vi "DAQmx.Prime AO.vi"(8 "error in (no error)":errorcluster, 11 "DAQmx in":refnum<class "DAQmx.lvclass">) -> (0 "error out":errorcluster, 3 "DAQmx out":refnum<class "DAQmx.lvclass">)   [LabVIEW 2019, in "DAQmx.lvclass"]
uses:
  DAQmx.lvclass
  DAQmx.lvclass/DAQmx.ctl
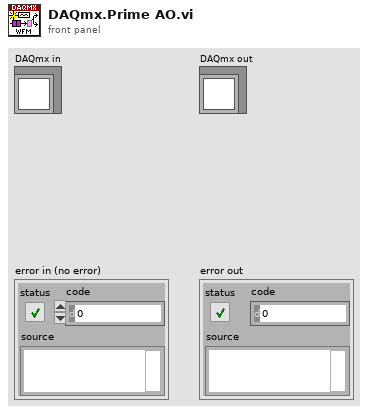
[diagram p1: front panel]
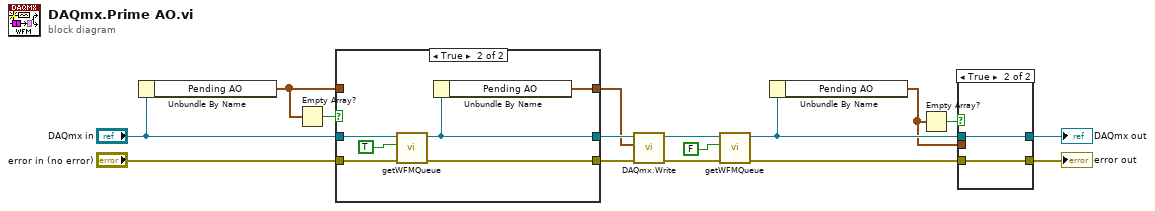
[diagram p0: block diagram]
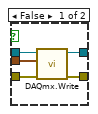
[diagram p2: hidden frame]
diagram:
  n1 = Unbundle By Name("DAQmx in") -> ("Pending AO"=w12:waveform(dbl)[])
  n2 = Empty Array?(array=w12) -> (empty?=w13:bool)
  n3 = case shown="True" w13 {
    tunnel: [w18 w21] -> w6
    tunnel: "DAQmx in" -> [w18 w25]
    tunnel: "error in (no error)" -> [w19 w24]
    tunnel: [w17 w20] -> w3
    tunnel: [w19 w22] -> w7
    tunnel: w12 -> [w17 _]
    frame False {
    }
    frame True {
      n4 = call "getWFMQueue.vi"("error in (no error)"=w24, "wait for min buffer?"=TRUE, "DAQmx in"=w25) -> ("error out"=w22:errorcluster, "DAQmx out"=w21:refnum<class "DAQmx.lvclass">)  [unwired: 6 in, 1 out]
      n5 = Unbundle By Name(w21) -> ("Pending AO"=w20:waveform(dbl)[])
    }
  }
  n6 = call "DAQmx.Write.vi"("error in (no error)"=w7, "AOwfm"=w3, "DAQmx in"=w6) -> ("error out"=w5:errorcluster, "DAQmx out"=w4:refnum<class "DAQmx.lvclass">)  [unwired: 6 in, 1 out]
  n7 = call "getWFMQueue.vi"("error in (no error)"=w5, "wait for min buffer?"=FALSE, "DAQmx in"=w4) -> ("error out"=w10:errorcluster, "DAQmx out"=w11:refnum<class "DAQmx.lvclass">)  [unwired: 6 in, 1 out]
  n8 = Unbundle By Name(w11) -> ("Pending AO"=w2:waveform(dbl)[])
  n9 = Empty Array?(array=w2) -> (empty?=w1:bool)
  n10 = case shown="True" w1 {
    tunnel: w11 -> [w30 w32]
    tunnel: w10 -> [w29 w31]
    tunnel: [w28 w32] -> w9
    tunnel: [w27 w31] -> w8
    tunnel: w2 -> [w26 _]
    frame False {
      n11 = call "DAQmx.Write.vi"("error in (no error)"=w29, "AOwfm"=w26, "DAQmx in"=w30) -> ("error out"=w27:errorcluster, "DAQmx out"=w28:refnum<class "DAQmx.lvclass">)  [unwired: 6 in, 1 out]
    }
    frame True {
    }
  }
  "DAQmx out" <- w9
  "error out" <- w8
